vi "Update Measurement List.vi"(8 "error in (no error)":errorcluster, 10 "List of Measurements":string[](array[string]), 11 "Operator UI in":refnum<class "Measurement UI.lvclass">) -> (0 "error out":errorcluster, 3 "Operator UI out":refnum<class "Measurement UI.lvclass">)   [LabVIEW 2015, in "Measurement UI.lvlib" / "Measurement UI.lvclass"]
uses:
  Measurement UI.lvclass
  Measurement UI.lvclass/Measurement UI.ctl
  Accessors/Read Measurement.vi
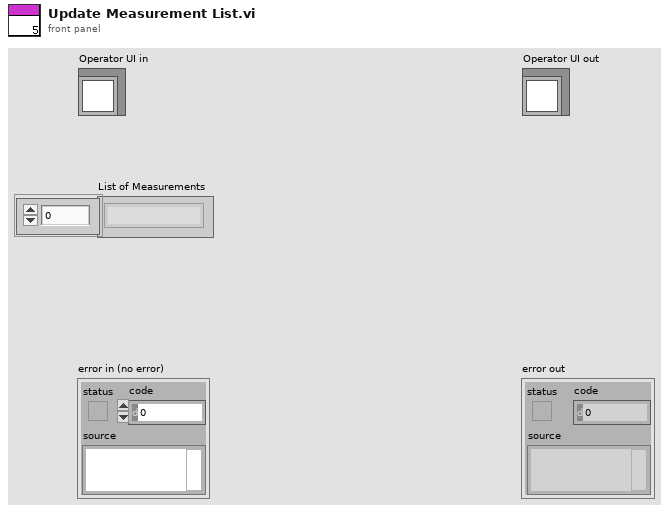
[diagram p1: front panel]
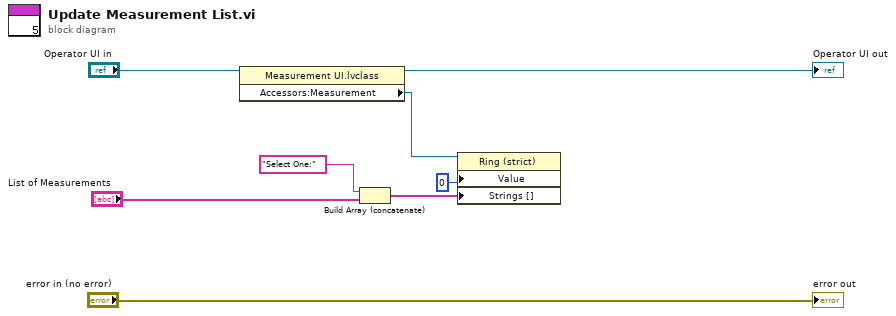
[diagram p0: block diagram]
diagram:
  n1 = property class="Measurement UI.lvclass"(reference="Operator UI in") -> (reference out=→"Operator UI out":refnum<class "Measurement UI.lvclass">, "Accessors:Measurement"=w1:refnum<vi>)  [unwired: 1 in, 1 out]
  n2 = Build Array (concatenate)("Select One:", "List of Measurements") -> (w5:string[])
  n3 = property class="Ring (strict)"(reference=w1, "Value"=u16 0, "Strings []"=w5) -> ()  [unwired: 1 in, 2 out]
  "error out" <- "error in (no error)"
